vi "Stop Process.vi"(8 "error in (no error)":errorcluster, 11 "DAQProc in":refnum<class "DAQProc.lvclass">) -> (0 "error out":errorcluster, 3 "DAQProc out":refnum<class "DAQProc.lvclass">)   [LabVIEW 2020, in "LAF2024Q2.lvlib" / "DAQProc.lvclass"]
uses:
  DAQProc.lvclass
  DAQProc.lvclass/DAQProc.ctl
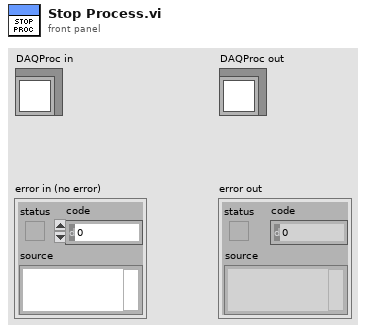
[diagram p1: front panel]
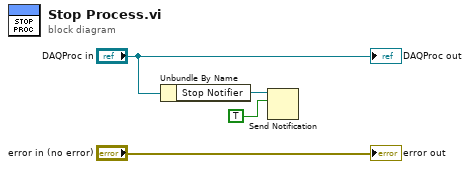
[diagram p0: block diagram]
diagram:
  n1 = Unbundle By Name("DAQProc in") -> ("Stop Notifier"=w2:refnum<notifier>)
  n2 = Send Notification(notification=TRUE, notifier=w2) -> ()  [unwired: 1 in, 2 out]
  "error out" <- "error in (no error)"
  "DAQProc out" <- "DAQProc in"
